vi "Actor Core.vi"(8 "error in":errorcluster, 11 "Test Caller Actor in":refnum<class "Test Caller Actor.lvclass">) -> (0 "error out":errorcluster, 3 "Actor out":refnum<class "Actor.lvclass">)   [LabVIEW 2023, in "Test Caller Actor.lvlib" / "Test Caller Actor.lvclass"]
doc: "(<B>Filename</B>: Actor Framework.lvlib:Actor.lvclass:Actor Core.vi)\n\nReceives messages to the actor, reacts to them, and initiates any error handling that may shut the actor down.\n\nDescendant classes may override this VI to append parallel tasks for the actor to complete while it handles messages. Overrides use the Call Parent Class Method node."
uses:
  Test Caller Actor.lvclass
  <vilib>/ActorFramework/Actor/Actor.lvclass
  Class Loader/Class Loader/Loading Progress.ctl
  Class Loader/Class Loader/Loading Method.ctl
  <vilib>/ActorFramework/Actor/Actor.lvclass/Actor.ctl
  <vilib>/ActorFramework/Message Enqueuer/Message Enqueuer.lvclass/Message Enqueuer.ctl
  Test Caller Actor.lvclass/Test Caller Actor.ctl
  <vilib>/ActorFramework/Message Enqueuer/Init from Existing Queue.vi
  <vilib>/ActorFramework/Message Enqueuer/Enqueue.vi
  <vilib>/ActorFramework/Stop Msg/Stop Msg.lvclass
  <vilib>/Utility/LVClass/Get LV Class Name.vi
  <resource>/AFDebug/Generate Trace for Message.vi
  <vilib>/ActorFramework/Message Priority Queue/Priority Enqueue.vi
  <vilib>/ActorFramework/Message Enqueuer/Message Enqueuer.lvclass
  <userlib>/_OpenG.lib/error/error.llb/openg_error.lvlib
  Class Loader/Class Loader Messages/Load Msg/Load Msg.lvclass
  Class Loader/Class Loader/Class Loader.lvclass
panel:
  in  "Loading Method":T1
  in  "Exit":bool
  in  "Load Concrete Classes":bool
  out "Class Names":string[](array[string])
  out "Load Complete":bool
  out "Loading Progress":T2 scale=0.0..100.0
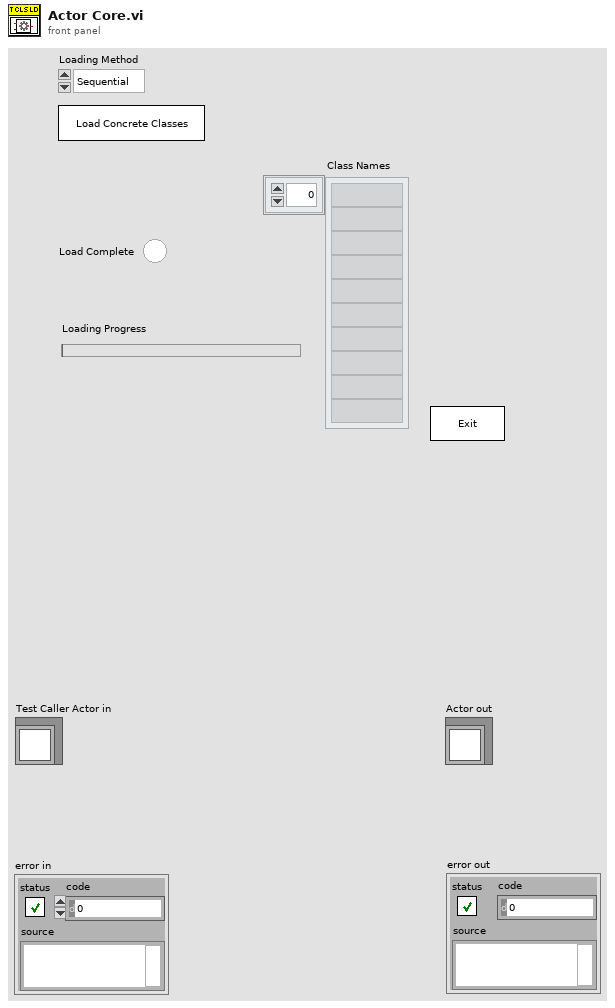
[diagram p1: front panel]
types:
  T1 = typedef "Class Loader.lvlib/Class Loader.lvclass/Loading Method.ctl" = enum16{"Sequential", "Parallel"}
  T2 = typedef "Class Loader.lvlib/Class Loader.lvclass/Loading Progress.ctl" = dbl
  T3 = enum32{"Invalid", "Standard", "Closed", "Hidden", "Minimized", "Maximized"}
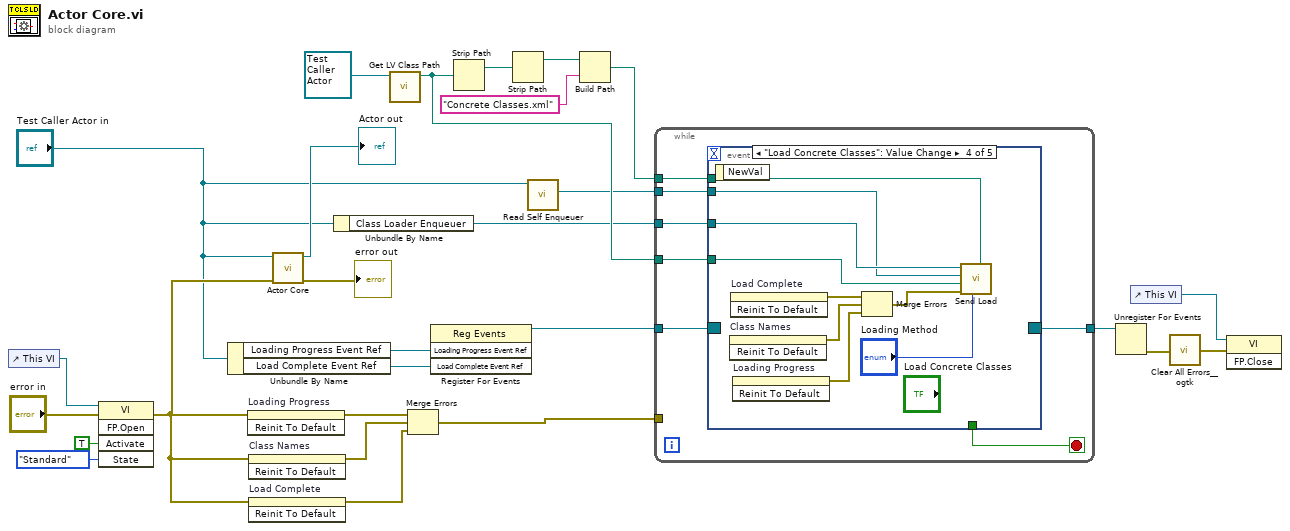
[diagram p0: block diagram]
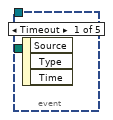
[diagram p2: hidden frame]
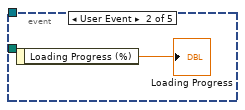
[diagram p3: hidden frame]
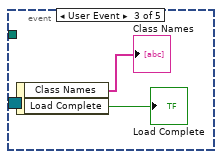
[diagram p4: hidden frame]
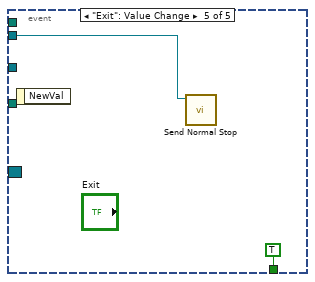
[diagram p5: hidden frame]
diagram:
  n1 = control-ref of="This VI"() -> (w9:refnum<vi>)
  n2 = invoke class="VI" method="FP.Open"(reference=w9, error in="error in", "Activate"=TRUE ("Activate?"), "State"=T3."Standard") -> (error out=w7:errorcluster)  [unwired: 1 in, 4 out]
  n3 = Unbundle By Name("Test Caller Actor in") -> ("Loading Progress Event Ref"=w26:refnum<user-event>, "Load Complete Event Ref"=w21:refnum<user-event>)
  n4 = invoke on="Loading Progress" class="Slide (strict)" method="Reinit To Default"(error in=w7) -> (error out=w24:errorcluster)  [unwired: 2 in, 2 out]
  n5 = invoke on="Class Names" class="Arr (strict)" method="Reinit To Default"(error in=w7) -> (error out=w19:errorcluster)  [unwired: 2 in, 2 out]
  n6 = invoke on="Load Complete" class="Bool (strict)" method="Reinit To Default"(error in=w7) -> (error out=w18:errorcluster)  [unwired: 2 in, 2 out]
  n7 = call-parent "Actor Core.vi"("error in"=w7, "Actor in"="Test Caller Actor in") -> ("error out"=→"error out":errorcluster, "Actor out"=→"Actor out":refnum<class "Actor.lvclass">)  [unwired: 8 in]
  n8 = Unbundle By Name("Test Caller Actor in") -> ("Class Loader Enqueuer"=w1:refnum<class "Message Enqueuer.lvclass">)
  n9 = call <vilib>:"Get LV Class Path.vi"("object"=refnum<class "Test Caller Actor.lvclass"> refnum ("Test Caller Actor.lvlib:Test Caller Actor.lvclass")) -> ("class path"=w11:path)  [unwired: 9 in, 1 out]
  n10 = Merge Errors(w24, w19, w18) -> (w20:errorcluster)
  n11 = register-events(w26, w21) -> (reference out=w25:refnum<event-registration>)  [unwired: 2 in, 1 out]
  n12 = Strip Path(path=w11) -> (stripped path=w15:path)  [unwired: 1 out]
  n13 = Strip Path(path=w15) -> (stripped path=w14:path)  [unwired: 1 out]
  n14 = call <vilib>:"Read Self Enqueuer.vi"("Actor"="Test Caller Actor in") -> ("Self Enqueuer"=w10:refnum<class "Message Enqueuer.lvclass">)  [unwired: 10 in]
  n15 = Build Path(base path=w14, name or relative path="Concrete Classes.xml") -> (appended path=w12:path)
  n16 = while {
    tunnel: w25 -> [w34]
    tunnel: w20 -> [_]
    tunnel: [w32] -> w23
    tunnel: w1 -> [w31]
    tunnel: w10 -> [w30]
    tunnel: w12 -> [w29]
    tunnel: w11 -> [w28]
    stop <- w33 stop-if-true
    n17 = event shown="[3] \"Load Concrete Classes\": Value Change" {
      selector: w34 -> [_ _ _ _ _]
      dyn-events: [_ _ _ _ _] -> w32
      timeout: _ -> [_ _ _ _ _]
      tunnel: [_ _ _ _ TRUE ("Exit")] -> w33
      tunnel: w31 -> [_ _ _ w43 _]
      tunnel: w30 -> [_ _ _ w41 w48]
      tunnel: w29 -> [_ _ _ w40 _]
      tunnel: w28 -> [_ _ _ w39 _]
      event Timeout {
        n18 = event-data() -> ()  [unwired: 1 in, 3 out]
      }
      event User Event {
        n19 = event-data() -> ("Loading Progress (%)"=→"Loading Progress":T2)  [unwired: 1 in]
      }
      event User Event {
        n20 = event-data() -> ("Class Names"=→"Class Names":string[], "Load Complete"=→"Load Complete":bool)  [unwired: 1 in]
      }
      event "Load Concrete Classes": Value Change {
        n21 = event-data() -> ()  [unwired: 1 in, 1 out]
        n22 = invoke on="Class Names" class="Arr (strict)" method="Reinit To Default"() -> (error out=w45:errorcluster)  [unwired: 3 in, 2 out]
        n23 = invoke on="Load Complete" class="Bool (strict)" method="Reinit To Default"() -> (error out=w46:errorcluster)  [unwired: 3 in, 2 out]
        n24 = invoke on="Loading Progress" class="Slide (strict)" method="Reinit To Default"() -> (error out=w44:errorcluster)  [unwired: 3 in, 2 out]
        n25 = Merge Errors(w46, w45, w44) -> (w42:errorcluster)
        n26 = call "Send Load.vi"("Class Relative Paths Path"=w40, "Loading Method"="Loading Method", "error in (no error)"=w42, "Reference Class Path"=w39, "Caller Enqueuer"=w41, "Message Enqueuer in"=w43) -> ()  [unwired: 4 in, 2 out]
      }
      event "Exit": Value Change {
        n27 = event-data() -> ()  [unwired: 1 in, 1 out]
        n28 = call <vilib>:"Send Normal Stop.vi"("Message Enqueuer"=w48) -> ()  [unwired: 10 in, 1 out]
      }
    }
  }
  n29 = Unregister For Events(event registration refnum=w23) -> (error out=w22:errorcluster)  [unwired: 1 in]
  n30 = control-ref of="This VI"() -> (w3:refnum<vi>)
  n31 = call <userlib>:"Clear All Errors__ogtk.vi"("Error In"=w22) -> ("Error Out"=w4:errorcluster)  [unwired: 3 in]
  n32 = invoke class="VI" method="FP.Close"(reference=w3, error in=w4) -> ()  [unwired: 1 in, 3 out]
